vi "Tree.vi"   [LabVIEW 8.6, in "ZTScopeM.lvlib"]
uses:
  ZTScopeM.lvlib
  Public/Upload Record (F32).vi
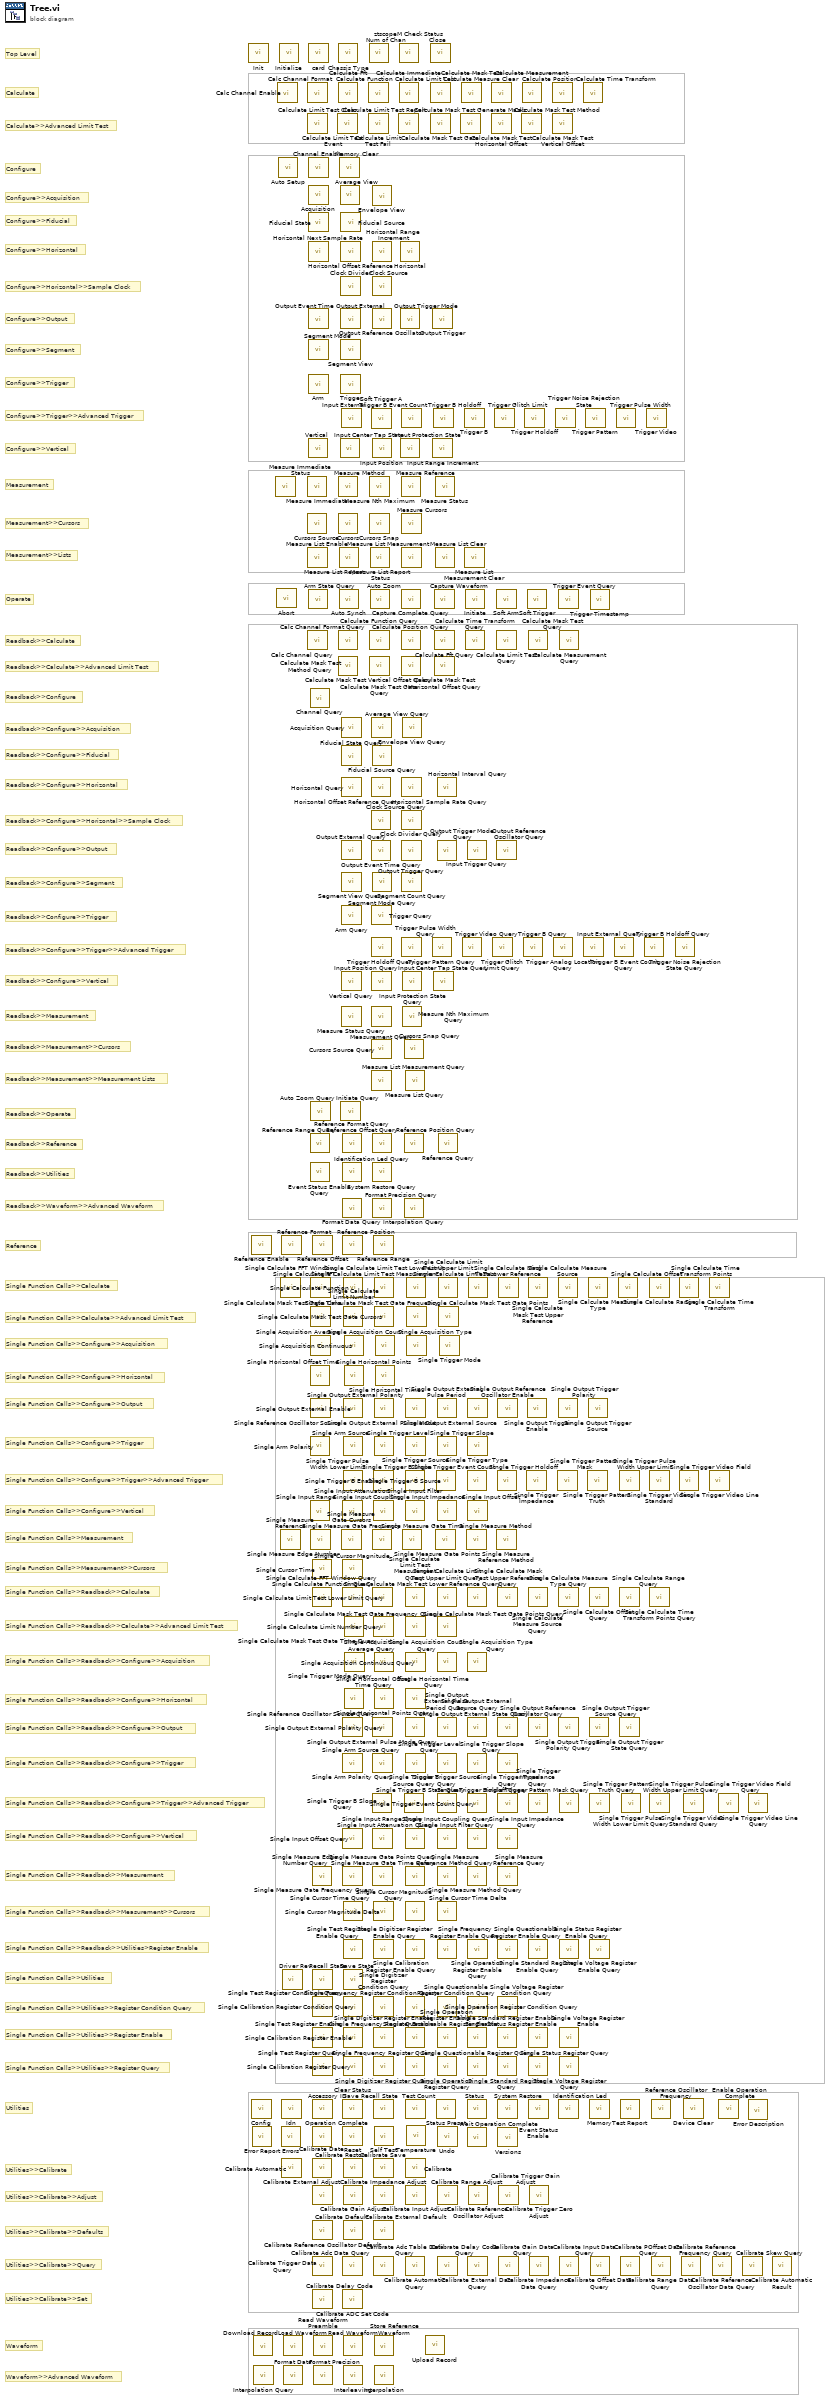
[diagram p0: block diagram]
diagram:
  # "Calculate>>Advanced Limit Test"
  # "Calculate"
  # "Operate"
  # "Measurement>>Lists"
  # "Measurement>>Cursors"
  # "Measurement"
  # "Configure>>Trigger"
  # "Configure>>Segment"
  # "Configure>>Fiducial"
  # "Configure"
  # "Top Level"
  # "Waveform>>Advanced Waveform"
  # "Waveform"
  # "Utilities>>Calibrate>>Set"
  # "Utilities>>Calibrate>>Query"
  # "Utilities>>Calibrate>>Defaults"
  # "Utilities>>Calibrate>>Adjust"
  # "Utilities>>Calibrate"
  # "Utilities"
  # "Single Function Calls>>Utilities>>Register Query"
  # "Single Function Calls>>Utilities>>Register Enable"
  # "Single Function Calls>>Utilities>>Register Condition Query"
  # "Single Function Calls>>Readback>>Measurement"
  # "Single Function Calls>>Utilities"
  # "Single Function Calls>>Readback>>Utilities>Register Enable"
  # "Single Function Calls>>Readback>>Measurement>>Cursors"
  # "Single Function Calls>>Readback>>Configure>>Vertical"
  # "Single Function Calls>>Readback>>Configure>>Trigger>>Advanced Trigger"
  # "Single Function Calls>>Readback>>Configure>>Trigger"
  # "Single Function Calls>>Readback>>Configure>>Output"
  # "Single Function Calls>>Readback>>Configure>>Horizontal"
  # "Single Function Calls>>Readback>>Configure>>Acquisition"
  # "Single Function Calls>>Readback>>Calculate>>Advanced Limit Test"
  # "Single Function Calls>>Readback>>Calculate"
  # "Single Function Calls>>Measurement>>Cursors"
  # "Single Function Calls>>Measurement"
  # "Single Function Calls>>Configure>>Vertical"
  # "Single Function Calls>>Configure>>Trigger>>Advanced Trigger"
  # "Single Function Calls>>Configure>>Trigger"
  # "Single Function Calls>>Configure>>Output"
  # "Single Function Calls>>Configure>>Horizontal"
  # "Single Function Calls>>Configure>>Acquisition"
  # "Single Function Calls>>Calculate>>Advanced Limit Test"
  # "Single Function Calls>>Calculate"
  # "Reference"
  # "Readback>>Waveform>>Advanced Waveform"
  # "Readback>>Utilities"
  # "Readback>>Reference"
  # "Readback>>Operate"
  # "Readback>>Measurement>>Measurement Lists"
  # "Readback>>Measurement"
  # "Readback>>Measurement>>Cursors"
  # "Readback>>Calculate>>Advanced Limit Test"
  # "Readback>>Calculate"
  # "Readback>>Configure>>Vertical"
  # "Readback>>Configure>>Output"
  # "Readback>>Configure>>Segment"
  # "Readback>>Configure>>Trigger"
  # "Readback>>Configure>>Trigger>>Advanced Trigger"
  # "Readback>>Configure>>Horizontal>>Sample Clock"
  # "Readback>>Configure>>Horizontal"
  # "Readback>>Configure>>Fiducial"
  # "Readback>>Configure>>Acquisition"
  # "Readback>>Configure"
  # "Configure>>Vertical"
  # "Configure>>Trigger>>Advanced Trigger"
  # "Configure>>Output"
  # "Configure>>Horizontal>>Sample Clock"
  # "Configure>>Horizontal"
  # "Configure>>Acquisition"
  n1 = call "Init.vi"() -> ()  [unwired: 8 in, 3 out]
  n2 = call "Reference Enable.vi"() -> ()  [unwired: 10 in, 2 out]
  n3 = call "Config.vi"() -> ()  [unwired: 9 in, 3 out]
  n4 = call "Error Report.vi"() -> ()  [unwired: 9 in, 3 out]
  n5 = call "Download Record.vi"() -> ()  [unwired: 9 in, 7 out]
  n6 = call "Interpolation Query.vi"() -> ()  [unwired: 9 in, 3 out]
  n7 = call "Measure Immediate Status.vi"() -> ()  [unwired: 8 in, 4 out]
  n8 = call "Abort.vi"() -> ()  [unwired: 10 in, 2 out]
  n9 = call "Calc Channel Enable.vi"() -> ()  [unwired: 10 in, 2 out]
  n10 = call "Auto Setup.vi"() -> ()  [unwired: 10 in, 2 out]
  n11 = call "Initialize.vi"() -> ()  [unwired: 10 in, 2 out]
  n12 = call "Single Calculate FFT Window.vi"() -> ()  [unwired: 10 in, 2 out]
  n13 = call "Single Measure Reference.vi"() -> ()  [unwired: 10 in, 2 out]
  n14 = call "Errors.vi"() -> ()  [unwired: 7 in, 4 out]
  n15 = call "Reference Format.vi"() -> ()  [unwired: 10 in, 2 out]
  n16 = call "Idn.vi"() -> ()  [unwired: 9 in, 3 out]
  n17 = call "Calibrate Automatic.vi"() -> ()  [unwired: 10 in, 2 out]
  n18 = call "Driver Rev.vi"() -> ()  [unwired: 9 in, 3 out]
  n19 = call "Load Waveform.vi"() -> ()  [unwired: 18 in, 2 out]
  n20 = call "Format Data.vi"() -> ()  [unwired: 10 in, 2 out]
  n21 = call "Measure Immediate.vi"() -> ()  [unwired: 9 in, 3 out]
  n22 = call "Cursors Source.vi"() -> ()  [unwired: 10 in, 2 out]
  n23 = call "Calc Channel Format.vi"() -> ()  [unwired: 10 in, 2 out]
  n24 = call "Calculate Limit Test Clear.vi"() -> ()  [unwired: 10 in, 2 out]
  n25 = call "Measure List Enable.vi"() -> ()  [unwired: 10 in, 2 out]
  n26 = call "Calc Channel Query.vi"() -> ()  [unwired: 9 in, 3 out]
  n27 = call "Vertical.vi"() -> ()  [unwired: 14 in, 2 out]
  n28 = call "Arm State Query.vi"() -> ()  [unwired: 9 in, 3 out]
  n29 = call "card.vi"() -> ()  [unwired: 4 in, 4 out]
  n30 = call "Channel Enable.vi"() -> ()  [unwired: 10 in, 2 out]
  n31 = call "Acquisition.vi"() -> ()  [unwired: 10 in, 2 out]
  n32 = call "Fiducial State.vi"() -> ()  [unwired: 10 in, 2 out]
  n33 = call "Horizontal Next Sample Rate.vi"() -> ()  [unwired: 8 in, 4 out]
  n34 = call "Output Event Time.vi"() -> ()  [unwired: 10 in, 2 out]
  n35 = call "Segment Mode.vi"() -> ()  [unwired: 10 in, 2 out]
  n36 = call "Arm.vi"() -> ()  [unwired: 10 in, 2 out]
  n37 = call "Channel Query.vi"() -> ()  [unwired: 9 in, 3 out]
  n38 = call "Reference Range Query.vi"() -> ()  [unwired: 9 in, 3 out]
  n39 = call "Event Status Enable Query.vi"() -> ()  [unwired: 8 in, 12 out]
  n40 = call "Single Horizontal Offset Time.vi"() -> ()  [unwired: 10 in, 2 out]
  n41 = call "Single Arm Polarity.vi"() -> ()  [unwired: 10 in, 2 out]
  n42 = call "Single Input Range.vi"() -> ()  [unwired: 10 in, 2 out]
  n43 = call "Auto Zoom Query.vi"() -> ()  [unwired: 8 in, 4 out]
  n44 = call "Single Calculate FFT.vi"() -> ()  [unwired: 10 in, 2 out]
  n45 = call "Single Calculate Mask Test Gate Time.vi"() -> ()  [unwired: 10 in, 2 out]
  n46 = call "Single Acquisition Average.vi"() -> ()  [unwired: 10 in, 2 out]
  n47 = call "Single Reference Oscillator Source.vi"() -> ()  [unwired: 10 in, 2 out]
  n48 = call "Single Measure Edge Number.vi"() -> ()  [unwired: 10 in, 2 out]
  n49 = call "Single Cursor Time.vi"() -> ()  [unwired: 10 in, 2 out]
  n50 = call "Single Calculate FFT Window Query.vi"() -> ()  [unwired: 9 in, 3 out]
  n51 = call "Single Measure Edge Number Query.vi"() -> ()  [unwired: 9 in, 3 out]
  n52 = call "Operation Complete.vi"() -> ()  [unwired: 9 in, 3 out]
  n53 = call "Calibrate Date.vi"() -> ()  [unwired: 6 in, 5 out]
  n54 = call "Reference Offset.vi"() -> ()  [unwired: 10 in, 2 out]
  n55 = call "Recall State.vi"() -> ()  [unwired: 10 in, 2 out]
  n56 = call "Single Test Register Condition Query.vi"() -> ()  [unwired: 9 in, 3 out]
  n57 = call "Single Test Register Enable.vi"() -> ()  [unwired: 10 in, 2 out]
  n58 = call "Single Test Register Query.vi"() -> ()  [unwired: 9 in, 3 out]
  n59 = call "Accessory ID.vi"() -> ()  [unwired: 9 in, 3 out]
  n60 = call "Calibrate External Adjust.vi"() -> ()  [unwired: 10 in, 2 out]
  n61 = call "Calibrate Reference Oscillator Default.vi"() -> ()  [unwired: 10 in, 2 out]
  n62 = call "Calibrate Trigger Data Query.vi"() -> ()  [unwired: 8 in, 4 out]
  n63 = call "Calibrate Delay Code.vi"() -> ()  [unwired: 10 in, 2 out]
  n64 = call "Read Waveform Preamble.vi"() -> ()  [unwired: 7 in, 9 out]
  n65 = call "Format Precision.vi"() -> ()  [unwired: 10 in, 2 out]
  n66 = call "Calculate Limit Test Event.vi"() -> ()  [unwired: 9 in, 3 out]
  n67 = call "Chassis Type.vi"() -> ()  [unwired: 9 in, 3 out]
  n68 = call "Calculate Fft.vi"() -> ()  [unwired: 10 in, 2 out]
  n69 = call "Measure Method.vi"() -> ()  [unwired: 10 in, 2 out]
  n70 = call "Cursors.vi"() -> ()  [unwired: 10 in, 2 out]
  n71 = call "Calc Channel Format Query.vi"() -> ()  [unwired: 9 in, 3 out]
  n72 = call "Calculate Mask Test Method Query.vi"() -> ()  [unwired: 9 in, 3 out]
  n73 = call "Measure List Report.vi"() -> ()  [unwired: 9 in, 3 out]
  n74 = call "Auto Synch.vi"() -> ()  [unwired: 10 in, 2 out]
  n75 = call "Memory Clear.vi"() -> ()  [unwired: 10 in, 2 out]
  n76 = call "Average View.vi"() -> ()  [unwired: 10 in, 2 out]
  n77 = call "Input Center Tap State.vi"() -> ()  [unwired: 10 in, 2 out]
  n78 = call "Fiducial Source.vi"() -> ()  [unwired: 10 in, 2 out]
  n79 = call "Horizontal Offset Reference.vi"() -> ()  [unwired: 10 in, 2 out]
  n80 = call "Clock Divider.vi"() -> ()  [unwired: 10 in, 2 out]
  n81 = call "Output External.vi"() -> ()  [unwired: 10 in, 2 out]
  n82 = call "Segment View.vi"() -> ()  [unwired: 10 in, 2 out]
  n83 = call "Trigger.vi"() -> ()  [unwired: 9 in, 2 out]
  n84 = call "Initiate Query.vi"() -> ()  [unwired: 9 in, 3 out]
  n85 = call "Input External.vi"() -> ()  [unwired: 10 in, 2 out]
  n86 = call "Acquisition Query.vi"() -> ()  [unwired: 6 in, 6 out]
  n87 = call "Fiducial State Query.vi"() -> ()  [unwired: 9 in, 3 out]
  n88 = call "Horizontal Query.vi"() -> ()  [unwired: 7 in, 5 out]
  n89 = call "Output External Query.vi"() -> ()  [unwired: 5 in, 7 out]
  n90 = call "Segment View Query.vi"() -> ()  [unwired: 9 in, 3 out]
  n91 = call "Arm Query.vi"() -> ()  [unwired: 7 in, 5 out]
  n92 = call "Vertical Query.vi"() -> ()  [unwired: 8 in, 8 out]
  n93 = call "Measure Status Query.vi"() -> ()  [unwired: 9 in, 3 out]
  n94 = call "Single Measure Gate Cursors.vi"() -> ()  [unwired: 10 in, 2 out]
  n95 = call "Reference Format Query.vi"() -> ()  [unwired: 9 in, 3 out]
  n96 = call "Identification Led Query.vi"() -> ()  [unwired: 9 in, 3 out]
  n97 = call "Format Data Query.vi"() -> ()  [unwired: 8 in, 4 out]
  n98 = call "Reference Position.vi"() -> ()  [unwired: 10 in, 2 out]
  n99 = call "Single Input Attenuation.vi"() -> ()  [unwired: 10 in, 2 out]
  n100 = call "Single Cursor Magnitude.vi"() -> ()  [unwired: 10 in, 2 out]
  n101 = call "Single Calculate Function Query.vi"() -> ()  [unwired: 7 in, 5 out]
  n102 = call "Single Reference Oscillator Source Query.vi"() -> ()  [unwired: 9 in, 3 out]
  n103 = call "Single Arm Polarity Query.vi"() -> ()  [unwired: 9 in, 3 out]
  n104 = call "Single Input Offset Query.vi"() -> ()  [unwired: 9 in, 3 out]
  n105 = call "Single Measure Gate Frequency Query.vi"() -> ()  [unwired: 8 in, 4 out]
  n106 = call "Clear Status.vi"() -> ()  [unwired: 10 in, 2 out]
  n107 = call "Reset.vi"() -> ()  [unwired: 10 in, 2 out]
  n108 = call "Calibrate Adc Data Query.vi"() -> ()  [unwired: 6 in, 6 out]
  n109 = call "Calibrate ADC Set Code.vi"() -> ()  [unwired: 10 in, 2 out]
  n110 = call "Single Calculate Function.vi"() -> ()  [unwired: 10 in, 2 out]
  n111 = call "Single Calculate Limit Number.vi"() -> ()  [unwired: 10 in, 2 out]
  n112 = call "Single Output External Enable.vi"() -> ()  [unwired: 10 in, 2 out]
  n113 = call "Single Arm Source.vi"() -> ()  [unwired: 10 in, 2 out]
  n114 = call "Single Trigger Pulse Width Lower Limit.vi"() -> ()  [unwired: 10 in, 2 out]
  n115 = call "Single Cursor Time Query.vi"() -> ()  [unwired: 9 in, 3 out]
  n116 = call "Single Test Register Enable Query.vi"() -> ()  [unwired: 9 in, 3 out]
  n117 = call "Save State.vi"() -> ()  [unwired: 10 in, 2 out]
  n118 = call "Single Calibration Register Condition Query.vi"() -> ()  [unwired: 9 in, 3 out]
  n119 = call "Single Calibration Register Enable.vi"() -> ()  [unwired: 10 in, 2 out]
  n120 = call "Single Calibration Register Query.vi"() -> ()  [unwired: 9 in, 3 out]
  n121 = call "Calibrate Restore.vi"() -> ()  [unwired: 10 in, 2 out]
  n122 = call "Calibrate Gain Adjust.vi"() -> ()  [unwired: 14 in, 2 out]
  n123 = call "Calibrate Default.vi"() -> ()  [unwired: 10 in, 2 out]
  n124 = call "Read Waveform.vi"() -> ()  [unwired: 8 in, 4 out]
  n125 = call "Interleaving.vi"() -> ()  [unwired: 9 in, 3 out]
  n126 = call "Single Acquisition Continuous.vi"() -> ()  [unwired: 10 in, 2 out]
  n127 = call "Single Horizontal Points.vi"() -> ()  [unwired: 10 in, 2 out]
  n128 = call "Single Calculate Mask Test Gate Time Query.vi"() -> ()  [unwired: 8 in, 4 out]
  n129 = call "Single Horizontal Offset Time Query.vi"() -> ()  [unwired: 9 in, 3 out]
  n130 = call "Single Trigger Mode Query.vi"() -> ()  [unwired: 9 in, 3 out]
  n131 = call "Calculate Function.vi"() -> ()  [unwired: 14 in, 2 out]
  n132 = call "Calculate Limit Test Fail.vi"() -> ()  [unwired: 9 in, 3 out]
  n133 = call "Num of Chan.vi"() -> ()  [unwired: 7 in, 5 out]
  n134 = call "Measure Nth Maximum.vi"() -> ()  [unwired: 10 in, 2 out]
  n135 = call "Cursors Snap.vi"() -> ()  [unwired: 10 in, 2 out]
  n136 = call "Calculate Function Query.vi"() -> ()  [unwired: 5 in, 7 out]
  n137 = call "Calculate Mask Test Gate Query.vi"() -> ()  [unwired: 8 in, 4 out]
  n138 = call "Measure List Report Status.vi"() -> ()  [unwired: 8 in, 4 out]
  n139 = call "Auto Zoom.vi"() -> ()  [unwired: 10 in, 2 out]
  n140 = call "Horizontal Offset Reference Query.vi"() -> ()  [unwired: 9 in, 3 out]
  n141 = call "Clock Source Query.vi"() -> ()  [unwired: 9 in, 3 out]
  n142 = call "Output Event Time Query.vi"() -> ()  [unwired: 9 in, 3 out]
  n143 = call "Soft Trigger A.vi"() -> ()  [unwired: 10 in, 2 out]
  n144 = call "Average View Query.vi"() -> ()  [unwired: 9 in, 3 out]
  n145 = call "Trigger Query.vi"() -> ()  [unwired: 6 in, 6 out]
  n146 = call "Trigger Holdoff Query.vi"() -> ()  [unwired: 8 in, 4 out]
  n147 = call "Input Position Query.vi"() -> ()  [unwired: 9 in, 3 out]
  n148 = call "Measurement Query.vi"() -> ()  [unwired: 6 in, 14 out]
  n149 = call "Cursors Source Query.vi"() -> ()  [unwired: 9 in, 3 out]
  n150 = call "Measure List Measurement Query.vi"() -> ()  [unwired: 8 in, 4 out]
  n151 = call "Envelope View.vi"() -> ()  [unwired: 10 in, 2 out]
  n152 = call "Horizontal Range Increment.vi"() -> ()  [unwired: 8 in, 4 out]
  n153 = call "Clock Source.vi"() -> ()  [unwired: 10 in, 2 out]
  n154 = call "Output Reference Oscillator.vi"() -> ()  [unwired: 10 in, 2 out]
  n155 = call "Input Position.vi"() -> ()  [unwired: 10 in, 2 out]
  n156 = call "Fiducial Source Query.vi"() -> ()  [unwired: 9 in, 3 out]
  n157 = call "Segment Mode Query.vi"() -> ()  [unwired: 9 in, 3 out]
  n158 = call "Reference Offset Query.vi"() -> ()  [unwired: 9 in, 3 out]
  n159 = call "System Restore Query.vi"() -> ()  [unwired: 7 in, 3 out]
  n160 = call "Format Precision Query.vi"() -> ()  [unwired: 8 in, 4 out]
  n161 = call "Single Measure Gate Frequency.vi"() -> ()  [unwired: 10 in, 2 out]
  n162 = call "Single Trigger B Slope Query.vi"() -> ()  [unwired: 9 in, 3 out]
  n163 = call "Single Calculate Limit Test Lower Limit Query.vi"() -> ()  [unwired: 9 in, 3 out]
  n164 = call "Single Output External Polarity Query.vi"() -> ()  [unwired: 9 in, 3 out]
  n165 = call "Single Arm Source Query.vi"() -> ()  [unwired: 9 in, 3 out]
  n166 = call "Single Input Range Query.vi"() -> ()  [unwired: 9 in, 3 out]
  n167 = call "Single Measure Gate Points Query.vi"() -> ()  [unwired: 8 in, 4 out]
  n168 = call "Reference Range.vi"() -> ()  [unwired: 10 in, 2 out]
  n169 = call "Single Trigger B Enable.vi"() -> ()  [unwired: 10 in, 2 out]
  n170 = call "Single Input Coupling.vi"() -> ()  [unwired: 10 in, 2 out]
  n171 = call "Single Calculate Limit Number Query.vi"() -> ()  [unwired: 9 in, 3 out]
  n172 = call "Single Cursor Magnitude Delta.vi"() -> ()  [unwired: 9 in, 3 out]
  n173 = call "Single Calibration Register Enable Query.vi"() -> ()  [unwired: 9 in, 3 out]
  n174 = call "Single Digitizer Register Condition Query.vi"() -> ()  [unwired: 9 in, 3 out]
  n175 = call "Single Digitizer Register Enable.vi"() -> ()  [unwired: 10 in, 2 out]
  n176 = call "Single Digitizer Register Query.vi"() -> ()  [unwired: 9 in, 3 out]
  n177 = call "Save Recall State.vi"() -> ()  [unwired: 10 in, 2 out]
  n178 = call "Calibrate Save.vi"() -> ()  [unwired: 10 in, 2 out]
  n179 = call "Calibrate Impedance Adjust.vi"() -> ()  [unwired: 10 in, 2 out]
  n180 = call "Calibrate External Default.vi"() -> ()  [unwired: 10 in, 2 out]
  n181 = call "Calibrate Adc Table Data Query.vi"() -> ()  [unwired: 8 in, 4 out]
  n182 = call "Single Calculate Limit Test Lower Limit.vi"() -> ()  [unwired: 10 in, 2 out]
  n183 = call "Single Calculate Mask Test Gate Cursors.vi"() -> ()  [unwired: 10 in, 2 out]
  n184 = call "Single Output External Polarity.vi"() -> ()  [unwired: 10 in, 2 out]
  n185 = call "Single Trigger Level.vi"() -> ()  [unwired: 10 in, 2 out]
  n186 = call "Single Acquisition Average Query.vi"() -> ()  [unwired: 9 in, 3 out]
  n187 = call "Single Horizontal Points Query.vi"() -> ()  [unwired: 9 in, 3 out]
  n188 = call "Self Test.vi"() -> ()  [unwired: 9 in, 3 out]
  n189 = call "Store Reference Waveform.vi"() -> ()  [unwired: 10 in, 2 out]
  n190 = call "Interpolation.vi"() -> ()  [unwired: 10 in, 2 out]
  n191 = call "Single Acquisition Count.vi"() -> ()  [unwired: 10 in, 2 out]
  n192 = call "Single Horizontal Time.vi"() -> ()  [unwired: 10 in, 2 out]
  n193 = call "Calculate Limit Test Report.vi"() -> ()  [unwired: 7 in, 9 out]
  n194 = call "ztscopeM Check Status.vi"() -> ()  [unwired: 6 in, 2 out]
  n195 = call "Calculate Immediate.vi"() -> ()  [unwired: 10 in, 2 out]
  n196 = call "Horizontal.vi"() -> ()  [unwired: 10 in, 2 out]
  n197 = call "Output Trigger Mode.vi"() -> ()  [unwired: 10 in, 2 out]
  n198 = call "Input Protection State.vi"() -> ()  [unwired: 10 in, 2 out]
  n199 = call "Measure Reference.vi"() -> ()  [unwired: 10 in, 2 out]
  n200 = call "Capture Complete Query.vi"() -> ()  [unwired: 9 in, 3 out]
  n201 = call "Calculate Position Query.vi"() -> ()  [unwired: 9 in, 3 out]
  n202 = call "Calculate Mask Test Vertical Offset Query.vi"() -> ()  [unwired: 9 in, 3 out]
  n203 = call "Trigger B Event Count.vi"() -> ()  [unwired: 10 in, 2 out]
  n204 = call "Measure Cursors.vi"() -> ()  [unwired: 8 in, 8 out]
  n205 = call "Measure List Measurement.vi"() -> ()  [unwired: 10 in, 2 out]
  n206 = call "Horizontal Sample Rate Query.vi"() -> ()  [unwired: 9 in, 3 out]
  n207 = call "Clock Divider Query.vi"() -> ()  [unwired: 9 in, 3 out]
  n208 = call "Output Trigger Query.vi"() -> ()  [unwired: 7 in, 5 out]
  n209 = call "Segment Count Query.vi"() -> ()  [unwired: 9 in, 3 out]
  n210 = call "Trigger Pulse Width Query.vi"() -> ()  [unwired: 5 in, 7 out]
  n211 = call "Envelope View Query.vi"() -> ()  [unwired: 9 in, 3 out]
  n212 = call "Input Protection State Query.vi"() -> ()  [unwired: 9 in, 3 out]
  n213 = call "Measure Nth Maximum Query.vi"() -> ()  [unwired: 9 in, 3 out]
  n214 = call "Single Measure Gate Points.vi"() -> ()  [unwired: 10 in, 2 out]
  n215 = call "Cursors Snap Query.vi"() -> ()  [unwired: 9 in, 3 out]
  n216 = call "Reference Position Query.vi"() -> ()  [unwired: 9 in, 3 out]
  n217 = call "Interpolation Query.vi"() -> ()  [unwired: 9 in, 3 out]
  n218 = call "Single Trigger B Source Query.vi"() -> ()  [unwired: 9 in, 3 out]
  n219 = call "Measure List Query.vi"() -> ()  [unwired: 9 in, 3 out]
  n220 = call "Single Trigger B Slope.vi"() -> ()  [unwired: 10 in, 2 out]
  n221 = call "Single Input Filter.vi"() -> ()  [unwired: 10 in, 2 out]
  n222 = call "Single Calculate Limit Test Measurement Query.vi"() -> ()  [unwired: 9 in, 3 out]
  n223 = call "Single Output External Pulse Mode Query.vi"() -> ()  [unwired: 9 in, 3 out]
  n224 = call "Single Input Attenuation Query.vi"() -> ()  [unwired: 9 in, 3 out]
  n225 = call "Single Measure Gate Time Query.vi"() -> ()  [unwired: 8 in, 4 out]
  n226 = call "Single Cursor Magnitude Query.vi"() -> ()  [unwired: 9 in, 3 out]
  n227 = call "Single Digitizer Register Enable Query.vi"() -> ()  [unwired: 9 in, 3 out]
  n228 = call "Single Frequency Register Condition Query.vi"() -> ()  [unwired: 9 in, 3 out]
  n229 = call "Single Frequency Register Enable.vi"() -> ()  [unwired: 10 in, 2 out]
  n230 = call "Single Frequency Register Query.vi"() -> ()  [unwired: 9 in, 3 out]
  n231 = call "Calibrate Automatic Query.vi"() -> ()  [unwired: 9 in, 3 out]
  n232 = call "Single Output External Pulse Mode.vi"() -> ()  [unwired: 10 in, 2 out]
  n233 = call "Single Trigger Source.vi"() -> ()  [unwired: 10 in, 2 out]
  n234 = call "Single Calculate Mask Test Gate Frequency Query.vi"() -> ()  [unwired: 8 in, 4 out]
  n235 = call "Single Acquisition Continuous Query.vi"() -> ()  [unwired: 9 in, 3 out]
  n236 = call "Single Horizontal Time Query.vi"() -> ()  [unwired: 9 in, 3 out]
  n237 = call "Single Trigger Level Query.vi"() -> ()  [unwired: 9 in, 3 out]
  n238 = call "Test Count.vi"() -> ()  [unwired: 9 in, 3 out]
  n239 = call "Calibrate.vi"() -> ()  [unwired: 9 in, 3 out]
  n240 = call "Calibrate Input Adjust.vi"() -> ()  [unwired: 10 in, 2 out]
  n241 = call "Single Calculate Limit Test Measurement.vi"() -> ()  [unwired: 10 in, 2 out]
  n242 = call "Temperature.vi"() -> ()  [unwired: 9 in, 3 out]
  n243 = call "Single Calculate Mask Test Gate Frequency.vi"() -> ()  [unwired: 10 in, 2 out]
  n244 = call "Single Acquisition Type.vi"() -> ()  [unwired: 10 in, 2 out]
  n245 = call-poly "Upload Record.vi"() -> ()  [unwired: 14 in, 2 out]
  n246 = call "Close.vi"() -> ()  [unwired: 11 in, 1 out]
  n247 = call "Calculate Limit Test.vi"() -> ()  [unwired: 14 in, 2 out]
  n248 = call "Calculate Mask Test Gate.vi"() -> ()  [unwired: 10 in, 2 out]
  n249 = call "Trigger Pattern Query.vi"() -> ()  [unwired: 7 in, 5 out]
  n250 = call "Output Trigger.vi"() -> ()  [unwired: 10 in, 2 out]
  n251 = call "Input Range Increment.vi"() -> ()  [unwired: 10 in, 2 out]
  n252 = call "Trigger B Holdoff.vi"() -> ()  [unwired: 10 in, 2 out]
  n253 = call "Input Center Tap State Query.vi"() -> ()  [unwired: 9 in, 3 out]
  n254 = call "Capture Waveform.vi"() -> ()  [unwired: 10 in, 2 out]
  n255 = call "Calculate Fft Query.vi"() -> ()  [unwired: 8 in, 4 out]
  n256 = call "Calculate Mask Test Horizontal Offset Query.vi"() -> ()  [unwired: 9 in, 3 out]
  n257 = call "Measure Status.vi"() -> ()  [unwired: 10 in, 2 out]
  n258 = call "Measure List Clear.vi"() -> ()  [unwired: 10 in, 2 out]
  n259 = call "Single Measure Gate Time.vi"() -> ()  [unwired: 10 in, 2 out]
  n260 = call "Single Trigger B Source.vi"() -> ()  [unwired: 10 in, 2 out]
  n261 = call "Status Preset.vi"() -> ()  [unwired: 10 in, 2 out]
  n262 = call "Horizontal Interval Query.vi"() -> ()  [unwired: 9 in, 3 out]
  n263 = call "Output Trigger Mode Query.vi"() -> ()  [unwired: 9 in, 3 out]
  n264 = call "Single Output External Pulse Period.vi"() -> ()  [unwired: 10 in, 2 out]
  n265 = call "Single Trigger Slope.vi"() -> ()  [unwired: 10 in, 2 out]
  n266 = call "Single Input Impedance.vi"() -> ()  [unwired: 10 in, 2 out]
  n267 = call "Single Calculate Limit Test Upper Limit Query.vi"() -> ()  [unwired: 9 in, 3 out]
  n268 = call "Single Calculate Mask Test Gate Points Query.vi"() -> ()  [unwired: 8 in, 4 out]
  n269 = call "Single Acquisition Count Query.vi"() -> ()  [unwired: 9 in, 3 out]
  n270 = call "Single Output External Pulse Period Query.vi"() -> ()  [unwired: 9 in, 3 out]
  n271 = call "Single Trigger Source Query.vi"() -> ()  [unwired: 9 in, 3 out]
  n272 = call "Single Trigger B State Query.vi"() -> ()  [unwired: 9 in, 3 out]
  n273 = call "Single Input Coupling Query.vi"() -> ()  [unwired: 9 in, 3 out]
  n274 = call "Single Measure Method Query.vi"() -> ()  [unwired: 9 in, 3 out]
  n275 = call "Single Cursor Time Delta.vi"() -> ()  [unwired: 9 in, 3 out]
  n276 = call "Single Frequency Register Enable Query.vi"() -> ()  [unwired: 9 in, 3 out]
  n277 = call "Single Operation Register Condition Query.vi"() -> ()  [unwired: 9 in, 3 out]
  n278 = call "Single Operation Register Enable.vi"() -> ()  [unwired: 10 in, 2 out]
  n279 = call "Single Operation Register Query.vi"() -> ()  [unwired: 9 in, 3 out]
  n280 = call "Undo.vi"() -> ()  [unwired: 10 in, 2 out]
  n281 = call "Calibrate Range Adjust.vi"() -> ()  [unwired: 10 in, 2 out]
  n282 = call "Calibrate Delay Code Query.vi"() -> ()  [unwired: 8 in, 3 out]
  n283 = call "Reference Query.vi"() -> ()  [unwired: 9 in, 3 out]
  n284 = call "Single Calculate Limit Test Upper Limit.vi"() -> ()  [unwired: 10 in, 2 out]
  n285 = call "Single Calculate Mask Test Gate Points.vi"() -> ()  [unwired: 10 in, 2 out]
  n286 = call "Single Trigger Mode.vi"() -> ()  [unwired: 10 in, 2 out]
  n287 = call "Calculate Mask Test Generate Masks.vi"() -> ()  [unwired: 9 in, 3 out]
  n288 = call "Calculate Mask Test.vi"() -> ()  [unwired: 10 in, 2 out]
  n289 = call "Trigger Video Query.vi"() -> ()  [unwired: 8 in, 8 out]
  n290 = call "Trigger B.vi"() -> ()  [unwired: 10 in, 2 out]
  n291 = call "Measure List Measurement Clear.vi"() -> ()  [unwired: 10 in, 2 out]
  n292 = call "Initiate.vi"() -> ()  [unwired: 10 in, 2 out]
  n293 = call "Calculate Time Transform Query.vi"() -> ()  [unwired: 8 in, 4 out]
  n294 = call "Single Measure Method.vi"() -> ()  [unwired: 10 in, 2 out]
  n295 = call "Input Trigger Query.vi"() -> ()  [unwired: 9 in, 3 out]
  n296 = call "Single Trigger Event Count.vi"() -> ()  [unwired: 10 in, 2 out]
  n297 = call "Single Calculate Mask Test Lower Reference Query.vi"() -> ()  [unwired: 9 in, 3 out]
  n298 = call "Single Acquisition Type Query.vi"() -> ()  [unwired: 9 in, 3 out]
  n299 = call "Single Output External Source Query.vi"() -> ()  [unwired: 9 in, 3 out]
  n300 = call "Single Trigger Slope Query.vi"() -> ()  [unwired: 9 in, 3 out]
  n301 = call "Single Trigger Event Count Query.vi"() -> ()  [unwired: 9 in, 3 out]
  n302 = call "Single Input Filter Query.vi"() -> ()  [unwired: 9 in, 3 out]
  n303 = call "Single Measure Reference Method Query.vi"() -> ()  [unwired: 9 in, 3 out]
  n304 = call "Single Questionable Register Enable.vi"() -> ()  [unwired: 10 in, 2 out]
  n305 = call "Single Questionable Register Query.vi"() -> ()  [unwired: 9 in, 3 out]
  n306 = call "Status.vi"() -> ()  [unwired: 8 in, 12 out]
  n307 = call "Wait Operation Complete.vi"() -> ()  [unwired: 10 in, 2 out]
  n308 = call "Single Output External Source.vi"() -> ()  [unwired: 10 in, 2 out]
  n309 = call "Single Trigger Type.vi"() -> ()  [unwired: 10 in, 2 out]
  n310 = call "Single Input Offset.vi"() -> ()  [unwired: 10 in, 2 out]
  n311 = call "Single Operation Register Enable Query.vi"() -> ()  [unwired: 9 in, 3 out]
  n312 = call "Single Questionable Register Condition Query.vi"() -> ()  [unwired: 9 in, 3 out]
  n313 = call "Calibrate External Data Query.vi"() -> ()  [unwired: 8 in, 4 out]
  n314 = call "Single Calculate Limit Test.vi"() -> ()  [unwired: 10 in, 2 out]
  n315 = call "Calibrate Reference Oscillator Adjust.vi"() -> ()  [unwired: 10 in, 2 out]
  n316 = call "Calculate Measure Clear.vi"() -> ()  [unwired: 10 in, 2 out]
  n317 = call "Calculate Mask Test Horizontal Offset.vi"() -> ()  [unwired: 10 in, 2 out]
  n318 = call "Trigger Glitch Limit Query.vi"() -> ()  [unwired: 9 in, 3 out]
  n319 = call "Trigger Glitch Limit.vi"() -> ()  [unwired: 10 in, 2 out]
  n320 = call "Soft Arm.vi"() -> ()  [unwired: 10 in, 2 out]
  n321 = call "Calculate Limit Test Query.vi"() -> ()  [unwired: 5 in, 7 out]
  n322 = call "Output Reference Oscillator Query.vi"() -> ()  [unwired: 8 in, 4 out]
  n323 = call "Single Measure Reference Method.vi"() -> ()  [unwired: 10 in, 2 out]
  n324 = call "Single Trigger Holdoff.vi"() -> ()  [unwired: 10 in, 2 out]
  n325 = call "Single Standard Register Enable.vi"() -> ()  [unwired: 10 in, 2 out]
  n326 = call "Single Standard Register Query.vi"() -> ()  [unwired: 9 in, 3 out]
  n327 = call "Single Output Reference Oscillator Enable.vi"() -> ()  [unwired: 10 in, 2 out]
  n328 = call "Single Calculate Mask Test Upper Reference Query.vi"() -> ()  [unwired: 9 in, 3 out]
  n329 = call "Single Output External State Query.vi"() -> ()  [unwired: 9 in, 3 out]
  n330 = call "Single Trigger Type Query.vi"() -> ()  [unwired: 9 in, 3 out]
  n331 = call "Single Trigger Holdoff Query.vi"() -> ()  [unwired: 9 in, 3 out]
  n332 = call "Single Input Impedance Query.vi"() -> ()  [unwired: 9 in, 3 out]
  n333 = call "Single Measure Reference Query.vi"() -> ()  [unwired: 7 in, 5 out]
  n334 = call "Single Questionable Register Enable Query.vi"() -> ()  [unwired: 9 in, 3 out]
  n335 = call "Single Voltage Register Condition Query.vi"() -> ()  [unwired: 9 in, 3 out]
  n336 = call "System Restore.vi"() -> ()  [unwired: 8 in, 2 out]
  n337 = call "Versions.vi"() -> ()  [unwired: 7 in, 5 out]
  n338 = call "Single Calculate Mask Test Lower Reference.vi"() -> ()  [unwired: 10 in, 2 out]
  n339 = call "Calibrate Trigger Gain Adjust.vi"() -> ()  [unwired: 10 in, 2 out]
  n340 = call "Calibrate Gain Data Query.vi"() -> ()  [unwired: 9 in, 3 out]
  n341 = call "Calculate Mask Test Method.vi"() -> ()  [unwired: 10 in, 2 out]
  n342 = call "Calculate Measurement.vi"() -> ()  [unwired: 10 in, 2 out]
  n343 = call "Trigger B Query.vi"() -> ()  [unwired: 6 in, 6 out]
  n344 = call "Trigger Holdoff.vi"() -> ()  [unwired: 10 in, 2 out]
  n345 = call "Single Trigger Impedance.vi"() -> ()  [unwired: 10 in, 2 out]
  n346 = call "Soft Trigger.vi"() -> ()  [unwired: 10 in, 2 out]
  n347 = call "Single Output Trigger Enable.vi"() -> ()  [unwired: 10 in, 2 out]
  n348 = call "Calculate Mask Test Query.vi"() -> ()  [unwired: 6 in, 6 out]
  n349 = call "Single Calculate Mask Test Upper Reference.vi"() -> ()  [unwired: 10 in, 2 out]
  n350 = call "Single Calculate Measure Source Query.vi"() -> ()  [unwired: 9 in, 3 out]
  n351 = call "Single Output Reference Oscillator Query.vi"() -> ()  [unwired: 9 in, 3 out]
  n352 = call "Single Trigger Impedance Query.vi"() -> ()  [unwired: 9 in, 3 out]
  n353 = call "Single Standard Register Enable Query.vi"() -> ()  [unwired: 9 in, 3 out]
  n354 = call "Single Status Register Enable.vi"() -> ()  [unwired: 10 in, 2 out]
  n355 = call "Single Status Register Query.vi"() -> ()  [unwired: 9 in, 3 out]
  n356 = call "Event Status Enable.vi"() -> ()  [unwired: 18 in, 2 out]
  n357 = call "Calibrate Trigger Zero Adjust.vi"() -> ()  [unwired: 10 in, 2 out]
  n358 = call "Calibrate Impedance Data Query.vi"() -> ()  [unwired: 8 in, 3 out]
  n359 = call "Calculate Position.vi"() -> ()  [unwired: 10 in, 2 out]
  n360 = call "Calculate Mask Test Vertical Offset.vi"() -> ()  [unwired: 10 in, 2 out]
  n361 = call "Trigger Analog Location Query.vi"() -> ()  [unwired: 9 in, 3 out]
  n362 = call "Trigger Noise Rejection State.vi"() -> ()  [unwired: 9 in, 2 out]
  n363 = call "Single Trigger Pattern Mask.vi"() -> ()  [unwired: 10 in, 2 out]
  n364 = call "Single Calculate Measure Source.vi"() -> ()  [unwired: 10 in, 2 out]
  n365 = call "Single Output Trigger Polarity.vi"() -> ()  [unwired: 10 in, 2 out]
  n366 = call "Trigger Event Query.vi"() -> ()  [unwired: 9 in, 3 out]
  n367 = call "Single Calculate Measure Type Query.vi"() -> ()  [unwired: 9 in, 3 out]
  n368 = call "Single Output Trigger Polarity Query.vi"() -> ()  [unwired: 9 in, 3 out]
  n369 = call "Identification Led.vi"() -> ()  [unwired: 10 in, 2 out]
  n370 = call "Calculate Measurement Query.vi"() -> ()  [unwired: 8 in, 4 out]
  n371 = call "Single Trigger Pattern Mask Query.vi"() -> ()  [unwired: 9 in, 3 out]
  n372 = call "Single Status Register Enable Query.vi"() -> ()  [unwired: 9 in, 3 out]
  n373 = call "Single Voltage Register Enable.vi"() -> ()  [unwired: 10 in, 2 out]
  n374 = call "Single Voltage Register Query.vi"() -> ()  [unwired: 9 in, 3 out]
  n375 = call "Calibrate Input Data Query.vi"() -> ()  [unwired: 8 in, 4 out]
  n376 = call "Calculate Time Transform.vi"() -> ()  [unwired: 10 in, 2 out]
  n377 = call "Input External Query.vi"() -> ()  [unwired: 8 in, 4 out]
  n378 = call "Trigger Pattern.vi"() -> ()  [unwired: 10 in, 2 out]
  n379 = call "Single Trigger Pattern Truth.vi"() -> ()  [unwired: 10 in, 2 out]
  n380 = call "Single Calculate Measure Type.vi"() -> ()  [unwired: 10 in, 2 out]
  n381 = call "Single Output Trigger Source.vi"() -> ()  [unwired: 10 in, 2 out]
  n382 = call "Single Calculate Offset Query.vi"() -> ()  [unwired: 9 in, 3 out]
  n383 = call "Single Output Trigger Source Query.vi"() -> ()  [unwired: 9 in, 3 out]
  n384 = call "Single Trigger Pattern Truth Query.vi"() -> ()  [unwired: 9 in, 3 out]
  n385 = call "Single Voltage Register Enable Query.vi"() -> ()  [unwired: 9 in, 3 out]
  n386 = call "Memory.vi"() -> ()  [unwired: 9 in, 3 out]
  n387 = call "Trigger Timestamp.vi"() -> ()  [unwired: 9 in, 3 out]
  n388 = call "Calibrate Offset Data Query.vi"() -> ()  [unwired: 8 in, 4 out]
  n389 = call "Trigger B Event Count Query.vi"() -> ()  [unwired: 9 in, 3 out]
  n390 = call "Trigger Pulse Width.vi"() -> ()  [unwired: 10 in, 2 out]
  n391 = call "Single Calculate Offset.vi"() -> ()  [unwired: 10 in, 2 out]
  n392 = call "Single Trigger Pulse Width Upper Limit.vi"() -> ()  [unwired: 10 in, 2 out]
  n393 = call "Single Calculate Range Query.vi"() -> ()  [unwired: 9 in, 3 out]
  n394 = call "Single Output Trigger State Query.vi"() -> ()  [unwired: 9 in, 3 out]
  n395 = call "Test Report.vi"() -> ()  [unwired: 9 in, 3 out]
  n396 = call "Calibrate POffset Data Query.vi"() -> ()  [unwired: 9 in, 3 out]
  n397 = call "Single Trigger Pulse Width Lower Limit Query.vi"() -> ()  [unwired: 9 in, 3 out]
  n398 = call "Trigger B Holdoff Query.vi"() -> ()  [unwired: 9 in, 3 out]
  n399 = call "Trigger Video.vi"() -> ()  [unwired: 10 in, 2 out]
  n400 = call "Single Calculate Range.vi"() -> ()  [unwired: 10 in, 2 out]
  n401 = call "Single Trigger Video Standard.vi"() -> ()  [unwired: 10 in, 2 out]
  n402 = call "Single Calculate Time Transform Points Query.vi"() -> ()  [unwired: 9 in, 3 out]
  n403 = call "Single Trigger Pulse Width Upper Limit Query.vi"() -> ()  [unwired: 9 in, 3 out]
  n404 = call "Reference Oscillator Frequency.vi"() -> ()  [unwired: 9 in, 3 out]
  n405 = call "Calibrate Range Data Query.vi"() -> ()  [unwired: 8 in, 4 out]
  n406 = call "Trigger Noise Rejection State Query.vi"() -> ()  [unwired: 7 in, 3 out]
  n407 = call "Single Calculate Time Transform Points.vi"() -> ()  [unwired: 10 in, 2 out]
  n408 = call "Single Trigger Video Field.vi"() -> ()  [unwired: 10 in, 2 out]
  n409 = call "Calibrate Reference Frequency Query.vi"() -> ()  [unwired: 9 in, 3 out]
  n410 = call "Single Trigger Video Standard Query.vi"() -> ()  [unwired: 9 in, 3 out]
  n411 = call "Device Clear.vi"() -> ()  [unwired: 10 in, 2 out]
  n412 = call "Single Calculate Time Transform.vi"() -> ()  [unwired: 10 in, 2 out]
  n413 = call "Single Trigger Video Line.vi"() -> ()  [unwired: 10 in, 2 out]
  n414 = call "Calibrate Reference Oscillator Data Query.vi"() -> ()  [unwired: 9 in, 3 out]
  n415 = call "Single Trigger Video Field Query.vi"() -> ()  [unwired: 9 in, 3 out]
  n416 = call "Enable Operation Complete.vi"() -> ()  [unwired: 10 in, 2 out]
  n417 = call "Calibrate Skew Query.vi"() -> ()  [unwired: 9 in, 3 out]
  n418 = call "Single Trigger Video Line Query.vi"() -> ()  [unwired: 9 in, 3 out]
  n419 = call "Error Description.vi"() -> ()  [unwired: 10 in, 2 out]
  n420 = call "Calibrate Automatic Result.vi"() -> ()  [unwired: 9 in, 3 out]
